vi "REQ Create CAN Database.vi"(8 "error in":errorcluster, 10 "Database Configuration":T1={"Interface"="CAN1", "CAN Cluster"={"Baud Rate"=125000, "Comment"="", "Name"="CAN_Cluster"}, "CAN Frame"={"Frame name"="frame1", "Identifier"=1, "Payload Length"=8, "Timing Type"=1, "Transmit Time"=0.0, "Extended Identifier?"=FALSE, "Comment"=""}, "Signal Cluster"={"Signal name"="signal", "Scaling Factor"=1.0, "Scaling Offset"=0.0, "Maximum Value"=256.0, "Minimum Value"=0.0, "Default Value"=0.0, "Unit"="V", "Start Bit"=0, "Number of Bits"=8, "Data Type"=1, "Byte Order"=0, "Comment"=""}, "Session Type (All Single Point)"=enum."Signal Input"} {"Signal Cluster"."Byte Order" items=["Little Endian", "Big Endian"]; "Signal Cluster"."Data Type" items=["Signed", "Unsigned", "IEEE Float"]; "CAN Frame"."Timing Type" items=["Cyclic Data", "Event Data", "Cyclic Remote", "Event Remote"]}) -> (0 "error out":errorcluster)   [LabVIEW 2021, in "CAN.lvlib"]
doc: "_____\nCreated using DQMH Event Scripter 6.1.0.128."
uses:
  CAN.lvlib
  Program Files (x86)/National Instruments/LabVIEW 2016/examples/nixnet/examples.llb/NI-XNET Example Control - Signal.ctl
  Program Files (x86)/National Instruments/LabVIEW 2016/examples/nixnet/examples.llb/NI-XNET Example Control - CAN Frame.ctl
  Program Files (x86)/National Instruments/LabVIEW 2016/examples/nixnet/examples.llb/NI-XNET Example Control - CAN Cluster.ctl
  CAN Database Configuration.ctl
  REQ Create CAN Database Argument--cluster.ctl
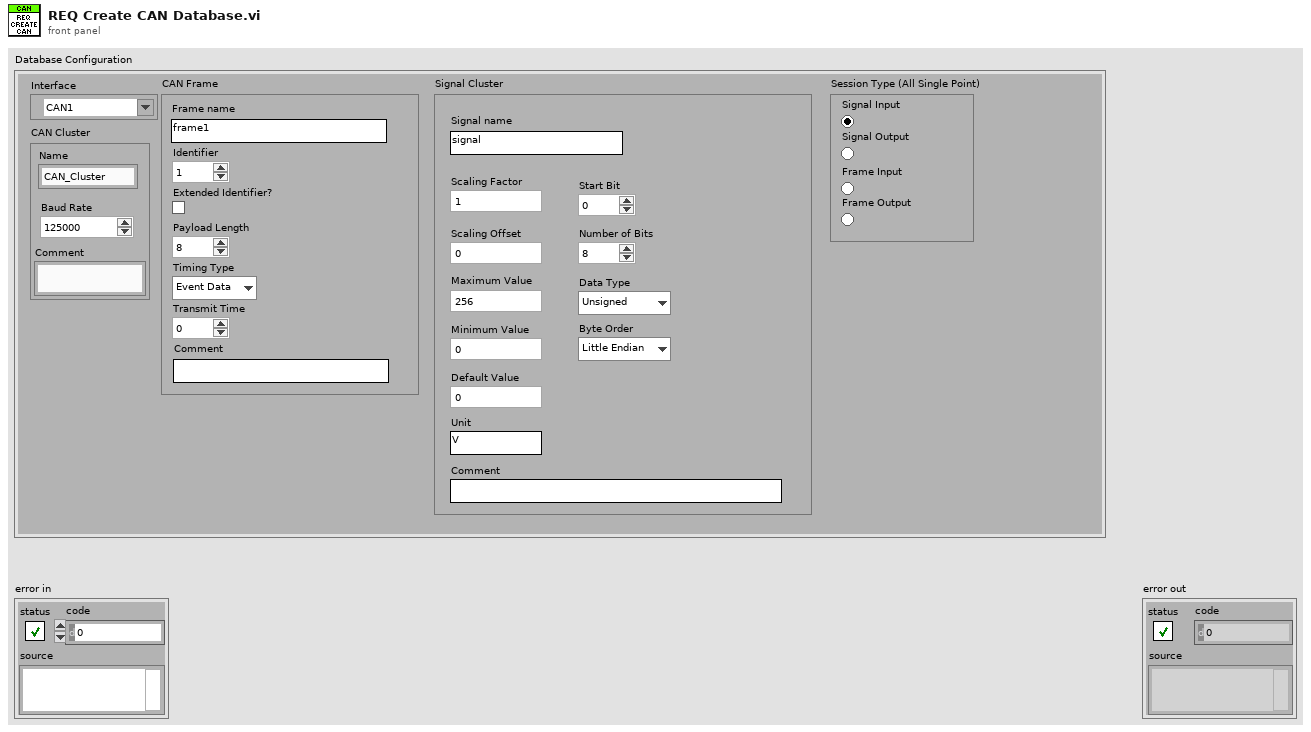
[diagram p1: front panel]
types:
  T1 = typedef "CAN.lvlib/CAN Database Configuration.ctl" = cluster{"Interface":refnum<k21>, "CAN Cluster":T2, "CAN Frame":T3, "Signal Cluster":T4, "Session Type (All Single Point)":enum32{"Signal Input", "Signal Output", "Frame Input", "Frame Output"}}
  T2 = typedef "NI-XNET Example Control - CAN Cluster.ctl" = cluster{"Baud Rate":u32, "Comment":string, "Name":string}
  T3 = typedef "NI-XNET Example Control - CAN Frame.ctl" = cluster{"Frame name":string, "Identifier":u32, "Payload Length":u32, "Timing Type":u32, "Transmit Time":dbl, "Extended Identifier?":bool, "Comment":string}
  T4 = typedef "NI-XNET Example Control - Signal.ctl" = cluster{"Signal name":string, "Scaling Factor":dbl, "Scaling Offset":dbl, "Maximum Value":dbl, "Minimum Value":dbl, "Default Value":dbl, "Unit":string, "Start Bit":u32, "Number of Bits":u32, "Data Type":u32, "Byte Order":u32, "Comment":string}
  T5 = typedef "CAN.lvlib/REQ Create CAN Database Argument--cluster.ctl" = cluster{"Database Configuration":T1}
  T6 = typedef "CAN.lvlib/Request Events--cluster.ctl" = cluster{"Stop Module":refnum<user-event>, "Show Panel":refnum<user-event>, "Hide Panel":refnum<user-event>, "Get Module Execution Status":refnum<user-event>, "Show Diagram":refnum<user-event>, "REQ Initialize Hardware":refnum<user-event>, "REQ Setup":refnum<user-event>, "REQ Get Channel Data":refnum<user-event>, "REQ CAN Data":refnum<user-event>, "REQ Close Ref":refnum<user-event>, "REQ Create CAN Database":refnum<user-event>}
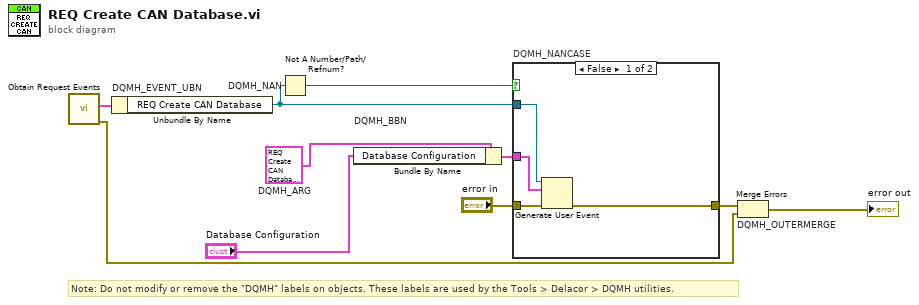
[diagram p0: block diagram]
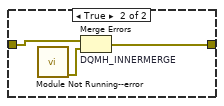
[diagram p2: hidden frame]
diagram:
  w4 = T5 {"Database Configuration"={"Interface"="CAN1", "CAN Cluster"={"Baud Rate"=125000, "Comment"="", "Name"="CAN_Cluster"}, "CAN Frame"={"Frame name"="frame1", "Identifier"=1, "Payload Length"=8, "Timing Type"=1, "Transmit Time"=0.0, "Extended Identifier?"=FALSE, "Comment"=""}, "Signal Cluster"={"Signal name"="signal", "Scaling Factor"=1.0, "Scaling Offset"=0.0, "Maximum Value"=256.0, "Minimum Value"=0.0, "Default Value"=0.0, "Unit"="V", "Start Bit"=0, "Number of Bits"=8, "Data Type"=1, "Byte Order"=0, "Comment"=""}, "Session Type (All Single Point)"=enum."Signal Input"}}  # DQMH_ARG
  # "Note: Do not modify or remove the \"DQMH\" labels on objects. These labels are used by the Tools > Delacor > DQMH utilities."
  n1 = call "Obtain Request Events.vi"() -> ("error out"=w2:errorcluster, "CAN Request Events"=w1:T6)  [unwired: 10 in]
  n2 = Unbundle By Name "DQMH_EVENT_UBN"(w1) -> ("REQ Create CAN Database"=w6:refnum<user-event>)
  n3 = Not A Number/Path/Refnum? "DQMH_NAN"(number/path/refnum=w6) -> (NaN/Path/Refnum?=w7:bool)
  n4 = Bundle By Name "DQMH_BBN"(cluster=w4, "Database Configuration"="Database Configuration") -> (w8:T5)
  n5 = case "DQMH_NANCASE" shown="False" w7 {
    tunnel: "error in" -> [w14 w17]
    tunnel: [w13 w16] -> w5
    tunnel: w6 -> [w12 _]
    tunnel: w8 -> [w11 _]
    frame False {
      n6 = Generate User Event(user event=w12, event data cluster=w11, error in=w14) -> (error out=w13:errorcluster)  [unwired: 1 in, 1 out]
    }
    frame True {
      n7 = call "Module Not Running--error.vi"() -> ("error out"=w15:errorcluster)  [unwired: 11 in]
      n8 = Merge Errors "DQMH_INNERMERGE"(w17, w15) -> (w16:errorcluster)
    }
  }
  n9 = Merge Errors "DQMH_OUTERMERGE"(w5, w2) -> (→"error out":errorcluster)
